vi "CopyOneBlock2D.vi"(8 "error in (no error)":errorcluster, 10 "block":u16) -> (0 "error out":errorcluster, 1 "data1":u16[][](array[numeric]), 2 "data0":u16[][](array[numeric]))   [LabVIEW 2015, in "ESLSCDLL.lvlib"]
uses:
  ESLSCDLL.lvlib
  Globals.vi
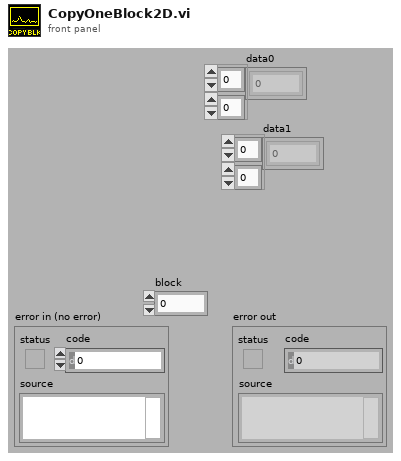
[diagram p1: front panel]
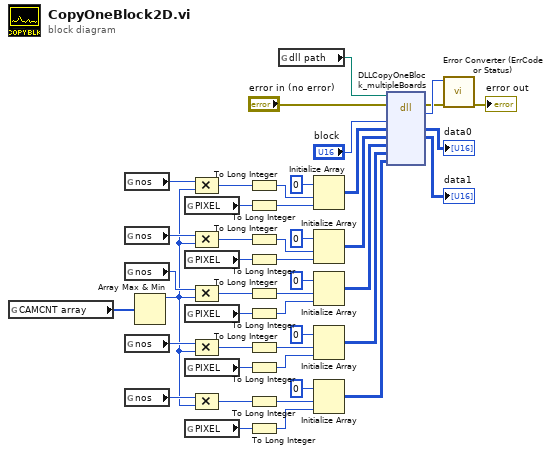
[diagram p0: block diagram]
diagram:
  n1 = global read "Globals.vi" "CAMCNT array"() -> (w33:u32[])
  n2 = global read "Globals.vi" "nos"() -> (w40:u32)
  n3 = global read "Globals.vi" "nos"() -> (w35:u32)
  n4 = global read "Globals.vi" "nos"() -> (w29:u32)
  n5 = global read "Globals.vi" "nos"() -> (w25:u32)
  n6 = global read "Globals.vi" "nos"() -> (w21:u32)
  n7 = Array Max & Min(array=w33) -> (max value=w20:u32)  [unwired: 3 out]
  n8 = global read "Globals.vi" "PIXEL"() -> (w16:u32)
  n9 = global read "Globals.vi" "PIXEL"() -> (w14:u32)
  n10 = global read "Globals.vi" "PIXEL"() -> (w11:u32)
  n11 = global read "Globals.vi" "PIXEL"() -> (w9:u32)
  n12 = global read "Globals.vi" "PIXEL"() -> (w7:u32)
  n13 = Compound Arithmetic op=MULTIPLY(w40, w20) -> (w41:u32)
  n14 = Compound Arithmetic op=MULTIPLY(w35, w20) -> (w36:u32)
  n15 = Compound Arithmetic op=MULTIPLY(w29, w20) -> (w30:u32)
  n16 = Compound Arithmetic op=MULTIPLY(w25, w20) -> (w26:u32)
  n17 = Compound Arithmetic op=MULTIPLY(w21, w20) -> (w22:u32)
  n18 = To Long Integer(number=w41) -> (32bit integer=w43:i32)
  n19 = To Long Integer(number=w16) -> (32bit integer=w15:i32)
  n20 = To Long Integer(number=w36) -> (32bit integer=w38:i32)
  n21 = To Long Integer(number=w14) -> (32bit integer=w13:i32)
  n22 = To Long Integer(number=w30) -> (32bit integer=w32:i32)
  n23 = To Long Integer(number=w11) -> (32bit integer=w12:i32)
  n24 = To Long Integer(number=w26) -> (32bit integer=w28:i32)
  n25 = To Long Integer(number=w9) -> (32bit integer=w10:i32)
  n26 = To Long Integer(number=w22) -> (32bit integer=w24:i32)
  n27 = To Long Integer(number=w7) -> (32bit integer=w8:i32)
  n28 = global read "Globals.vi" "dll path"() -> (w1:path)
  n29 = Initialize Array(u16 0, w43, w15) -> (w39:u16[][])
  n30 = Initialize Array(u16 0, w38, w13) -> (w34:u16[][])
  n31 = Initialize Array(u16 0, w32, w12) -> (w19:u16[][])
  n32 = Initialize Array(u16 0, w28, w10) -> (w18:u16[][])
  n33 = Initialize Array(u16 0, w24, w8) -> (w17:u16[][])
  n34 = dll-call lib="C:/ENTW/PCIE/LV64/board.vis/ESLSCDLL.dll" fn="DLLCopyOneBlock_multipleBoards" ("lwlscdll.dll:DLLReadLongS0")(path in=w1, error in="error in (no error)", "block"="block", "pdest0"=w39, "pdest1"=w34, "pdest2"=w19, "pdest3"=w18, "pdest4"=w17) -> (error out=w3:errorcluster, "es_status_codes"=w4:i32, "pdest0"=→"data0":u16[][], "pdest1"=→"data1":u16[][])  [unwired: 5 in, 1 out]
  n35 = call "Error Converter (ErrCode or Status).vi"("error in (no error)"=w3, "error code"=w4) -> ("error out"=→"error out":errorcluster)  [unwired: 9 in]
